vi "Post Pruning Decision Trees.vi"() -> ()   [LabVIEW 2020]
doc: "The DecisionTreeClassifier provides parameters such as min_samples_leaf and max_depth to prevent a tree from overfiting. Cost complexity pruning provides another option to control the size of a tree. In DecisionTreeClassifier, this pruning technique is parameterized by the cost complexity parameter, ccp_alpha. Greater values of ccp_alpha increase the number of nodes pruned. Here we only show the effect of ccp_alpha on regularizing the trees and how to choose a ccp_alpha based on validation scores."
uses:
  Model/Supervised/Tree/DecisionTreeClassifier/DecisionTreeClassifier.lvclass
  C:/Users/cipop/TDF Dropbox/2_Technologies de France/1 - Services et Etudes/PLAIY/2 - DEV/PLAIYLAB/code/Model/Model.lvclass
  C:/Users/cipop/TDF Dropbox/2_Technologies de France/1 - Services et Etudes/PLAIY/2 - DEV/PLAIYLAB/code/Model/Supervised/Tree/Tree.lvclass
  Model/Supervised/Tree/DecisionTreeClassifier/Controls/decision_tree_classifier_params.ctl
  Model/Supervised/Tree/DecisionTreeClassifier/DecisionTreeClassifier.vi
panel:
  out "Plot 2":cluster{"X":dbl[], "Y":dbl[]}[](graph) caption="Accuracy vs alpha for training and testing sets"
  out "Plot":cluster{"X":dbl[], "Y":dbl[]}(graph) caption="Total impurity vs effective alpha for training set"
  in  "Local":T1
  out "error out":errorcluster
  in  "error in":errorcluster
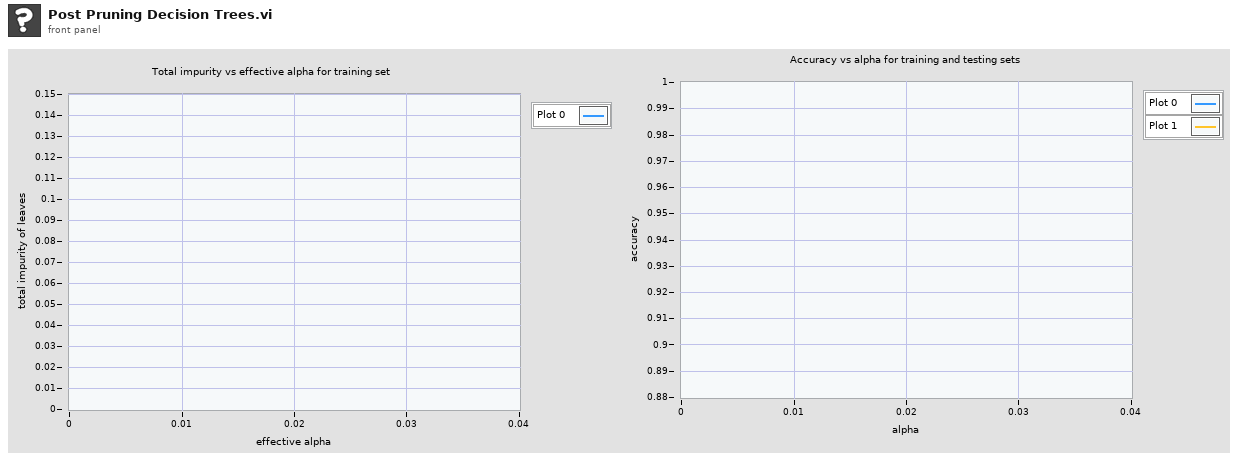
[diagram p1: front panel]
types:
  T1 = cluster{"X Test":dbl[][], "X Train":dbl[][], "Y Test":dbl[], "Y Train":dbl[], "ccp_alphas":dbl[], "impurities":dbl[], "DecisionTreeClassifier":refnum<class "DecisionTreeClassifier.lvclass">, "train_score":dbl[], "test_score":dbl[]}
  T2 = cluster{"test_size":dbl, "train_size":dbl, "random_state":i32, "shuffle":bool, "stratify":string[]}
  T3 = typedef "decision_tree_classifier_params.ctl" = cluster{"criterion":string, "splitter":string, "max_depth":cluster{"max_depth_type":string, "max_depth_int":dbl}, "min_samples_split":dbl, "min_samples_leaf":dbl, "min_weight_fraction_leaf":dbl, "max_features":cluster{"max_features_type":string, "max_features_int":dbl, "max_features_float":dbl}, "random_state":dbl, "max_leaf_nodes":cluster{"max_leaf_nodes_type":string, "max_leaf_nodes_int":dbl}, "min_impurity_decrease":dbl, "class_weight":cluster{"class_weight_type":string, "class_weight_dict":string}, "ccp_alpha":dbl}
  T4 = cluster{" 4DArray":cluster{"1":string[][], "2":string[][]}[], " 3DArray":cluster{"Tableau":string[][]}[], "Sparse Matrix 2DArray":string[][], " 2DArray":string[][], " 1DArray":string[]}
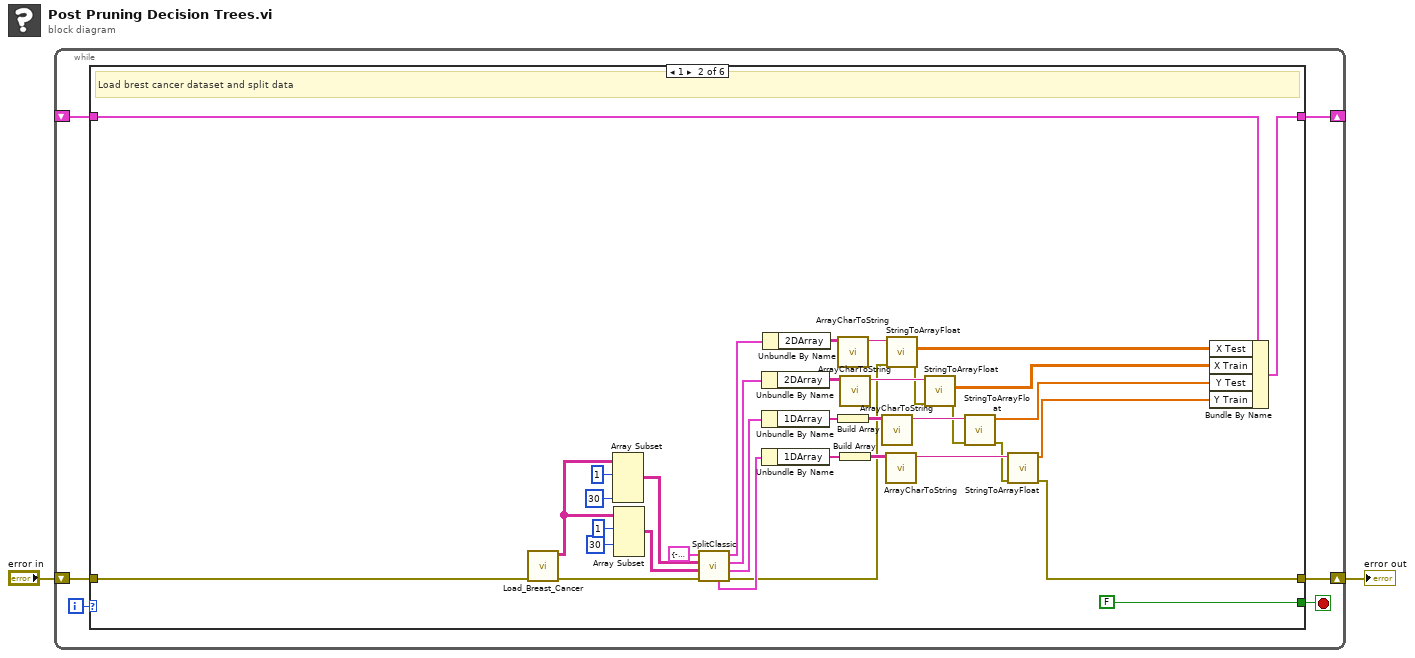
[diagram p0: block diagram]
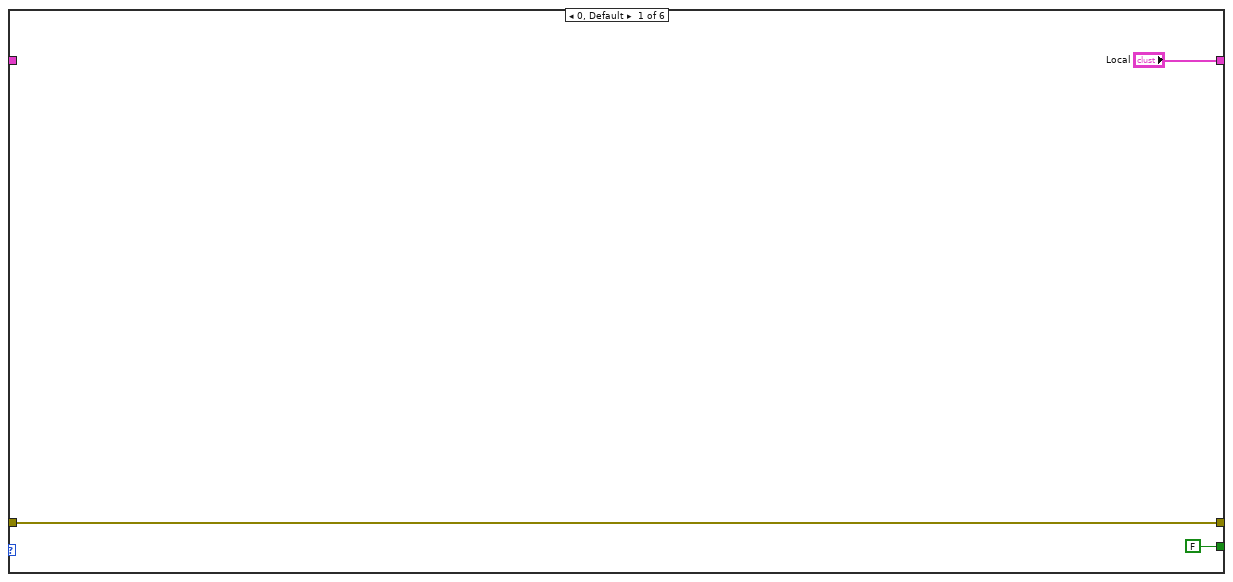
[diagram p2: hidden frame]
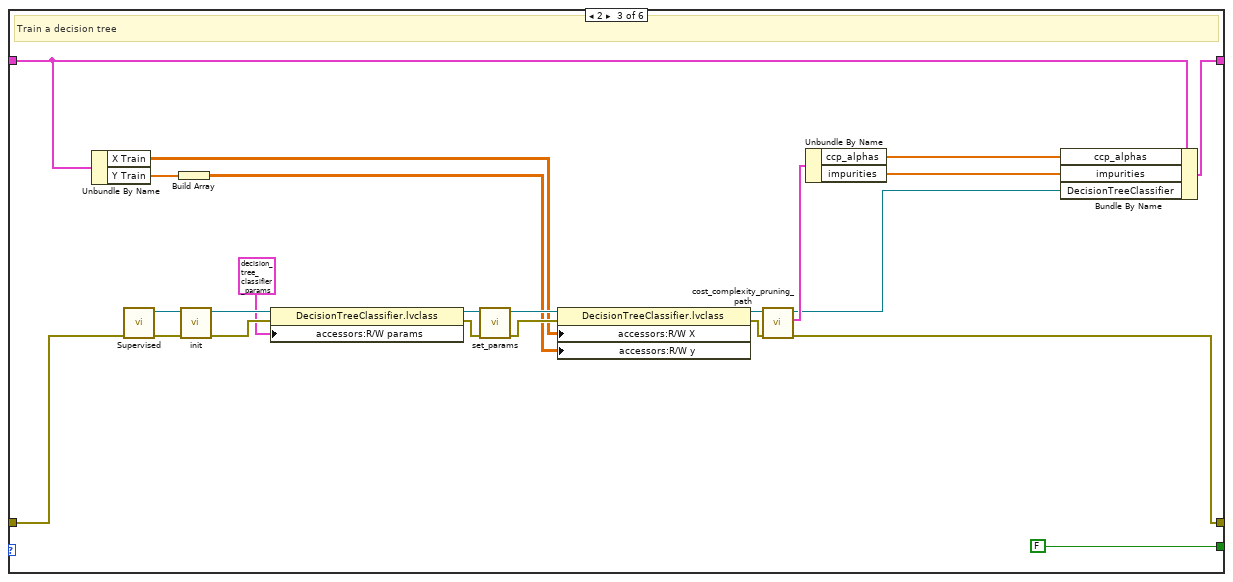
[diagram p3: hidden frame]
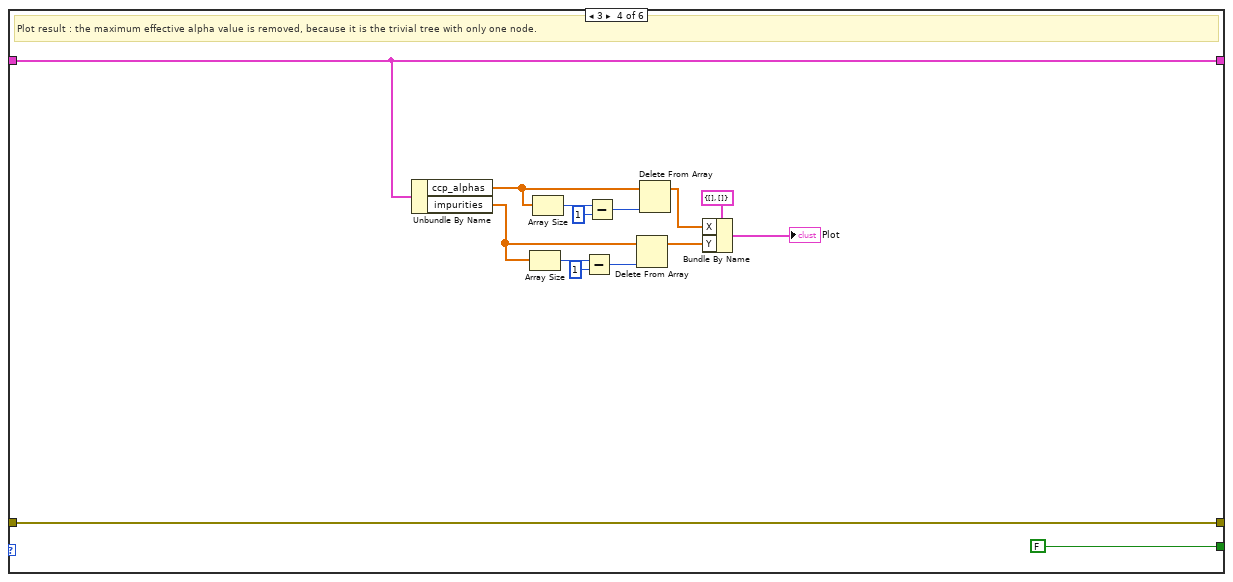
[diagram p4: hidden frame]
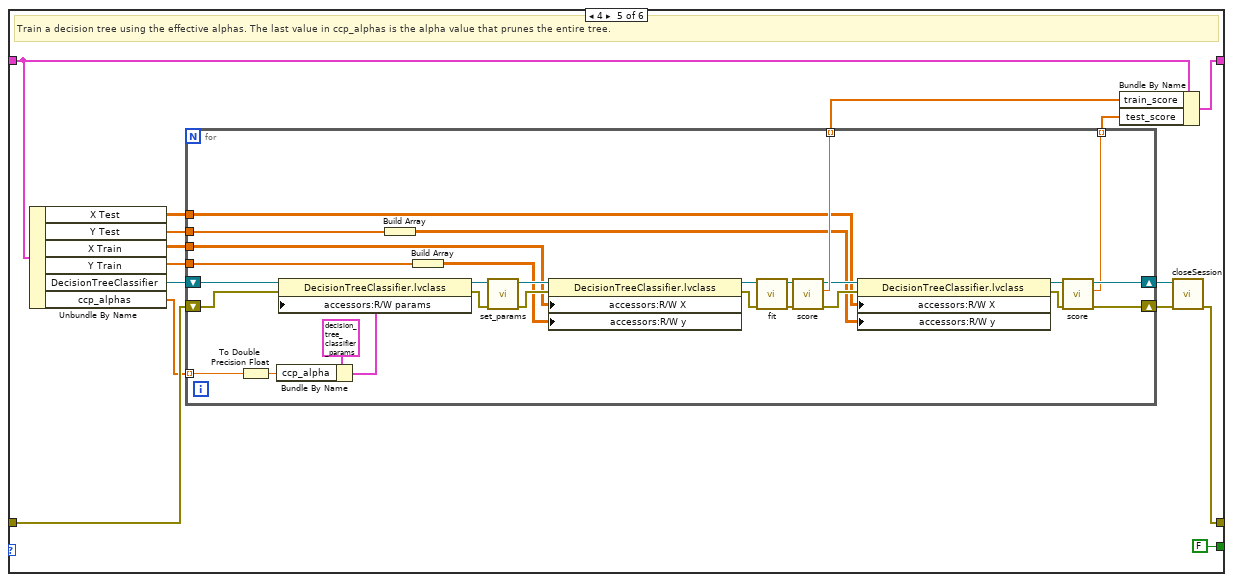
[diagram p5: hidden frame]
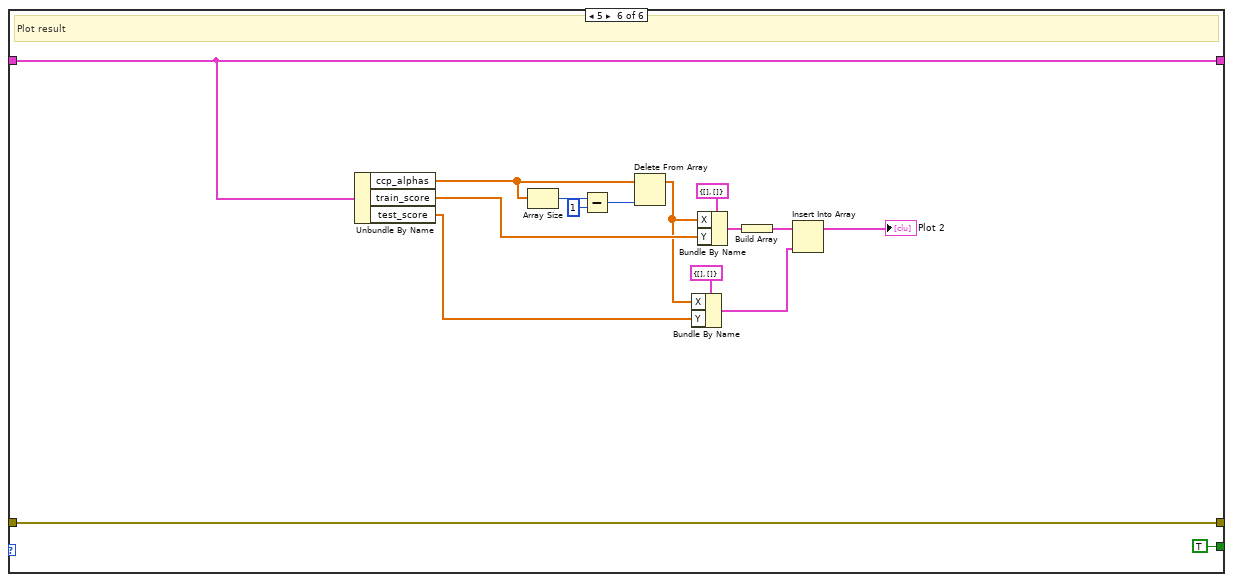
[diagram p6: hidden frame]
diagram:
  n1 = while {
    shift-right: [w6] -> w1
    shift-left: "error in" -> [w7]
    shift-right: [w5] -> _
    shift-left: _ -> [w4]
    i -> [w8]
    stop <- w3 stop-if-true
    n2 = case shown="1" w8 {
      tunnel: w7 -> [w10 w47 w62 w72 w93 w143]
      tunnel: [w10 w12 w48 w72 w95 w143] -> w6
      tunnel: ["Local" w37 w53 w73 w88 w136] -> w5
      tunnel: w4 -> [_ w38 w54 w73 w89 w136]
      tunnel: [FALSE FALSE FALSE FALSE FALSE TRUE] -> w3
      frame 0, Default {
      }
      frame 1 {
        # "Load brest cancer dataset and split data"
        n3 = call "Load_Breast_Cancer.vi"("error in"=w47) -> ("error out"=w35:errorcluster, "Tableau"=w39:string[][])  [unwired: 9 in]
        n4 = Array Subset(array=w39, index (row)=1 ("index"), length (col)=30 ("length")) -> (w32:string[][])  [unwired: 2 in]
        n5 = Array Subset(array=w39, index (row)=1 ("index"), index (col)=30 ("index")) -> (w33:string[][])  [unwired: 2 in]
        n6 = call "SplitClassic.vi"("error in (no error)"=w35, "Y"=w33, "X"=w32, "TestTrain"=T2 {"test_size"=-1.0, "train_size"=-1.0, "random_state"=0, "shuffle"=TRUE, "stratify"=[]}) -> ("error out"=w16:errorcluster, "Y_Test"=w26:T4, "X_Train"=w29:T4, "X_Test"=w31:T4, "Y_Train"=w21:T4)  [unwired: 3 in]
        n7 = Unbundle By Name(w29) -> ("2DArray"=w28:string[][])
        n8 = Unbundle By Name(w26) -> ("1DArray"=w25:string[])
        n9 = Unbundle By Name(w21) -> ("1DArray"=w20:string[])
        n10 = Unbundle By Name(w31) -> ("2DArray"=w30:string[][])
        n11 = call "ArrayCharToString.vi"("TAB"=w30) -> ("Instruction"=w41:string)  [unwired: 10 in]
        n12 = Build Array(w25) -> (w24:string[][])
        n13 = call "ArrayCharToString.vi"("TAB"=w28) -> ("Instruction"=w40:string)  [unwired: 10 in]
        n14 = Build Array(w20) -> (w19:string[][])
        n15 = call "ArrayCharToString.vi"("TAB"=w24) -> ("Instruction"=w23:string)  [unwired: 10 in]
        n16 = call "ArrayCharToString.vi"("TAB"=w19) -> ("Instruction"=w18:string)  [unwired: 10 in]
        n17 = call "StringToArrayFloat.vi"("entrée d'erreur (pas d'erreur)"=w16, "Return value"=w41) -> ("error IO"=w15:errorcluster, "2DArray"=w36:dbl[][])  [unwired: 7 in, 1 out]
        n18 = call "StringToArrayFloat.vi"("entrée d'erreur (pas d'erreur)"=w15, "Return value"=w40) -> ("error IO"=w14:errorcluster, "2DArray"=w27:dbl[][])  [unwired: 7 in, 1 out]
        n19 = call "StringToArrayFloat.vi"("entrée d'erreur (pas d'erreur)"=w14, "Return value"=w23) -> ("error IO"=w13:errorcluster, "1DArray"=w22:dbl[])  [unwired: 7 in, 1 out]
        n20 = call "StringToArrayFloat.vi"("entrée d'erreur (pas d'erreur)"=w13, "Return value"=w18) -> ("error IO"=w12:errorcluster, "1DArray"=w17:dbl[])  [unwired: 7 in, 1 out]
        n21 = Bundle By Name(cluster=w38, "X Test"=w36, "X Train"=w27, "Y Test"=w22, "Y Train"=w17) -> (w37:T1)
      }
      frame 2 {
        # "Train a decision tree"
        n22 = Unbundle By Name(w54) -> ("X Train"=w60:dbl[][], "Y Train"=w59:dbl[])
        n23 = call-poly "Supervised.vi"("error in"=w62) -> ("error out"=w63:errorcluster, "out"=w64:refnum<class "DecisionTreeClassifier.lvclass">)  [unwired: 9 in]
        n24 = Build Array(w59) -> (w58:dbl[][])
        n25 = call-dynamic "init.vi"("error in (no error)"=w63, "Model en entrée"=w64) -> ("error out"=w65:errorcluster, "Model en sortie"=w69:refnum<class "DecisionTreeClassifier.lvclass">)  [unwired: 8 in]
        n26 = property class="DecisionTreeClassifier.lvclass"(reference=w69, error in=w65, "accessors:R/W params"=T3 {"criterion"="gini", "splitter"="best", "max_depth"={"max_depth_type"="None", "max_depth_int"=0.0}, "min_samples_split"=2.0, "min_samples_leaf"=1.0, "min_weight_fraction_leaf"=0.0, "max_features"={"max_features_type"="None", "max_features_int"=0.0, "max_features_float"=0.0}, "random_state"=0.0, "max_leaf_nodes"={"max_leaf_nodes_type"="None", "max_leaf_nodes_int"=100.0}, "min_impurity_decrease"=0.0, "class_weight"={"class_weight_type"="None", "class_weight_dict"="{0:1.1, 2:1.5, 2:0.6}"}, "ccp_alpha"=0.0} ("R/W params")) -> (reference out=w68:refnum<class "DecisionTreeClassifier.lvclass">, error out=w50:errorcluster)
        n27 = call-dynamic "set_params.vi"("error in (no error)"=w50, "DecisionTreeClassifier.lvclass 2"=w68) -> ("error out"=w66:errorcluster, "DecisionTreeClassifier.lvclass"=w67:refnum<class "DecisionTreeClassifier.lvclass">)  [unwired: 8 in]
        n28 = property class="DecisionTreeClassifier.lvclass"(reference=w67, error in=w66, "accessors:R/W X"=w60, "accessors:R/W y"=w58) -> (reference out=w57:refnum<class "DecisionTreeClassifier.lvclass">, error out=w56:errorcluster)
        n29 = call-dynamic "cost_complexity_pruning_path.vi"("error in (no error)"=w56, "Tree.lvclass"=w57) -> ("error out"=w48:errorcluster, "out"=w55:cluster{"ccp_alphas":dbl[], "impurities":dbl[]}, "Tree.lvclass 2"=w49:refnum<class "DecisionTreeClassifier.lvclass">)  [unwired: 7 in]
        n30 = Unbundle By Name(w55) -> ("ccp_alphas"=w52:dbl[], "impurities"=w51:dbl[])
        n31 = Bundle By Name(cluster=w54, "ccp_alphas"=w52, "impurities"=w51, "DecisionTreeClassifier"=w49) -> (w53:T1)
      }
      frame 3 {
        # "Plot result : the maximum effective alpha value is removed, because it is the trivial tree with only one node."
        n32 = Unbundle By Name(w73) -> ("ccp_alphas"=w85:dbl[], "impurities"=w78:dbl[])
        n33 = Array Size(array=w78) -> (size(s)=w79:i32)
        n34 = Array Size(array=w85) -> (size(s)=w84:i32)
        n35 = Subtract(x=w79, y=1) -> (x-y=w80:i32)
        n36 = Subtract(x=w84, y=1) -> (x-y=w83:i32)
        n37 = Delete From Array(array=w78, index=w80) -> (array with subset deleted=w75:dbl[])  [unwired: 1 in, 1 out]
        n38 = Delete From Array(array=w85, index=w83) -> (array with subset deleted=w76:dbl[])  [unwired: 1 in, 1 out]
        n39 = Bundle By Name(cluster=cluster{"X":dbl[], "Y":dbl[]} {"X"=[], "Y"=[]} ("Cluster"), "X"=w76, "Y"=w75) -> (→"Plot":cluster{"X":dbl[], "Y":dbl[]})
      }
      frame 4 {
        # "Train a decision tree using the effective alphas. The last value in ccp_alphas is the alpha value that prunes the entire tree."
        n40 = Unbundle By Name(w89) -> ("X Test"=w92:dbl[][], "Y Test"=w91:dbl[], "X Train"=w99:dbl[][], "Y Train"=w98:dbl[], "DecisionTreeClassifier"=w100:refnum<class "DecisionTreeClassifier.lvclass">, "ccp_alphas"=w90:dbl[])
        n41 = for {
          tunnel: w99 -> [w121]
          tunnel: w98 -> [w120]
          shift-right: [w107] -> w97
          shift-left: w100 -> [w124]
          shift-right: [w106] -> w96
          shift-left: w93 -> [w115]
          tunnel: [w112] -> w87 mode=indexing
          tunnel: [w105] -> w86 mode=indexing
          tunnel: w90 -> [w101] mode=indexing
          tunnel: w92 -> [w104]
          tunnel: w91 -> [w103]
          n42 = To Double Precision Float(number=w101) -> (double precision float=w116:dbl)
          n43 = Bundle By Name(cluster=T3 {"criterion"="gini", "splitter"="best", "max_depth"={"max_depth_type"="None", "max_depth_int"=0.0}, "min_samples_split"=2.0, "min_samples_leaf"=1.0, "min_weight_fraction_leaf"=0.0, "max_features"={"max_features_type"="None", "max_features_int"=0.0, "max_features_float"=0.0}, "random_state"=0.0, "max_leaf_nodes"={"max_leaf_nodes_type"="None", "max_leaf_nodes_int"=100.0}, "min_impurity_decrease"=0.0, "class_weight"={"class_weight_type"="None", "class_weight_dict"="{0:1.1, 2:1.5, 2:0.6}"}, "ccp_alpha"=0.0} ("R/W params"), "ccp_alpha"=w116) -> (w122:T3)
          n44 = property class="DecisionTreeClassifier.lvclass"(reference=w124, error in=w115, "accessors:R/W params"=w122) -> (reference out=w128:refnum<class "DecisionTreeClassifier.lvclass">, error out=w125:errorcluster)
          n45 = Build Array(w103) -> (w102:dbl[][])
          n46 = Build Array(w120) -> (w119:dbl[][])
          n47 = call-dynamic "set_params.vi"("error in (no error)"=w125, "DecisionTreeClassifier.lvclass 2"=w128) -> ("error out"=w126:errorcluster, "DecisionTreeClassifier.lvclass"=w127:refnum<class "DecisionTreeClassifier.lvclass">)  [unwired: 8 in]
          n48 = property class="DecisionTreeClassifier.lvclass"(reference=w127, error in=w126, "accessors:R/W X"=w121, "accessors:R/W y"=w119) -> (reference out=w118:refnum<class "DecisionTreeClassifier.lvclass">, error out=w117:errorcluster)
          n49 = call-dynamic "fit.vi"("error in (no error)"=w117, "Tree.lvclass 2"=w118) -> ("error out"=w113:errorcluster, "Tree.lvclass"=w114:refnum<class "DecisionTreeClassifier.lvclass">)  [unwired: 8 in]
          n50 = call-dynamic "score.vi"("error in (no error)"=w113, "Tree.lvclass 2"=w114) -> ("error out"=w110:errorcluster, "score"=w112:dbl, "Tree.lvclass"=w111:refnum<class "DecisionTreeClassifier.lvclass">)  [unwired: 7 in]
          n51 = property class="DecisionTreeClassifier.lvclass"(reference=w111, error in=w110, "accessors:R/W X"=w104, "accessors:R/W y"=w102) -> (reference out=w108:refnum<class "DecisionTreeClassifier.lvclass">, error out=w109:errorcluster)
          n52 = call-dynamic "score.vi"("error in (no error)"=w109, "Tree.lvclass 2"=w108) -> ("error out"=w106:errorcluster, "score"=w105:dbl, "Tree.lvclass"=w107:refnum<class "DecisionTreeClassifier.lvclass">)  [unwired: 7 in]
        }
        n53 = Bundle By Name(cluster=w89, "train_score"=w87, "test_score"=w86) -> (w88:T1)
        n54 = call-dynamic "closeSession.vi"("error in"=w96, "Python en entrée"=w97) -> ("error out"=w95:errorcluster)  [unwired: 8 in, 1 out]
      }
      frame 5 {
        # "Plot result"
        n55 = Unbundle By Name(w136) -> ("ccp_alphas"=w142:dbl[], "train_score"=w135:dbl[], "test_score"=w130:dbl[])
        n56 = Array Size(array=w142) -> (size(s)=w141:i32)
        n57 = Subtract(x=w141, y=1) -> (x-y=w140:i32)
        n58 = Delete From Array(array=w142, index=w140) -> (array with subset deleted=w131:dbl[])  [unwired: 1 in, 1 out]
        n59 = Bundle By Name(cluster=cluster{"X":dbl[], "Y":dbl[]} {"X"=[], "Y"=[]} ("Cluster"), "X"=w131, "Y"=w130) -> (w129:cluster{"X":dbl[], "Y":dbl[]})
        n60 = Bundle By Name(cluster=cluster{"X":dbl[], "Y":dbl[]} {"X"=[], "Y"=[]} ("Cluster"), "X"=w131, "Y"=w135) -> (w137:cluster{"X":dbl[], "Y":dbl[]})
        n61 = Build Array(w137) -> (w134:cluster{"X":dbl[], "Y":dbl[]}[])
        n62 = Insert Into Array(array=w134, new element=w129) -> (→"Plot 2":cluster{"X":dbl[], "Y":dbl[]}[])  [unwired: 1 in]
      }
    }
  }
  "error out" <- w1
